vi "State_FGV.vi"() -> ()   [LabVIEW 2017]
panel:
  out "error out":errorcluster
  in  "error in (no error)":errorcluster
  out "OUT 5":bool
  out "OUT 4":bool
  out "OUT 3":bool
  out "OUT 2":bool
  out "OUT":bool
  in  "IN 5":bool
  in  "IN 4":bool
  in  "IN 3":bool
  in  "IN 2":bool
  in  "IN":bool
  in  "Enum":enum16{"SET", "GET"}(ring)
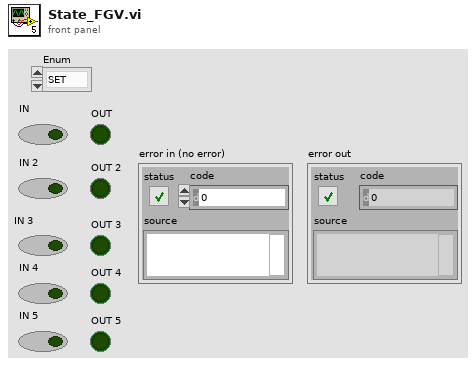
[diagram p1: front panel]
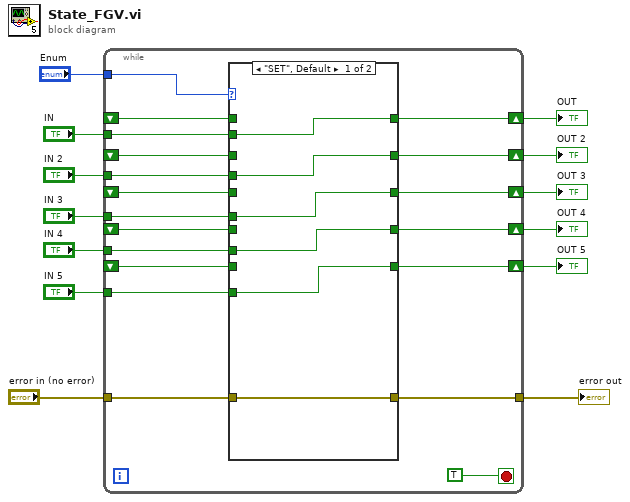
[diagram p0: block diagram]
diagram:
  n1 = while {
    shift-right: [w29] -> w5
    shift-left: _ -> [w19]
    shift-right: [w27] -> w4
    shift-left: _ -> [w18]
    shift-right: [w25] -> w3
    shift-left: _ -> [w17]
    shift-right: [w23] -> w2
    shift-left: _ -> [w16]
    shift-right: [w21] -> w1
    shift-left: _ -> [w15]
    tunnel: "Enum" -> [w32]
    tunnel: [w31] -> w12
    tunnel: "error in (no error)" -> [w30]
    tunnel: "IN" -> [w28]
    tunnel: "IN 2" -> [w26]
    tunnel: "IN 3" -> [w24]
    tunnel: "IN 4" -> [w22]
    tunnel: "IN 5" -> [w20]
    stop <- TRUE stop-if-true
    n2 = case shown="\"SET\", Default" w32 {
      tunnel: [w38 w44] -> w31
      tunnel: w30 -> [w38 w44]
      tunnel: [w37 w43] -> w29
      tunnel: w28 -> [w37 _]
      tunnel: [w36 w42] -> w27
      tunnel: w26 -> [w36 _]
      tunnel: [w35 w41] -> w25
      tunnel: w24 -> [w35 _]
      tunnel: [w34 w40] -> w23
      tunnel: w22 -> [w34 _]
      tunnel: [w33 w39] -> w21
      tunnel: w20 -> [w33 _]
      tunnel: w19 -> [_ w43]
      tunnel: w18 -> [_ w42]
      tunnel: w17 -> [_ w41]
      tunnel: w16 -> [_ w40]
      tunnel: w15 -> [_ w39]
      frame "SET", Default {
      }
      frame "GET" {
      }
    }
  }
  "OUT" <- w5
  "OUT 2" <- w4
  "OUT 3" <- w3
  "OUT 4" <- w2
  "OUT 5" <- w1
  "error out" <- w12
